vi "findCom.vi"(8 "error in (no error)":errorcluster, 11 "GiaoTiep in":refnum<class "GiaoTiepUART.lvclass">) -> (0 "error out":errorcluster, 3 "GiaoTiep out":refnum<class "GiaoTiepUART.lvclass">)   [LabVIEW 2014, in "LibraryGcode.lvlib" / "GiaoTiepUART.lvclass"]
uses:
  libraryGcode/ClassUART/GiaoTiepUART.lvclass
  <vilib>/Instr/_visa.llb/VISA Find Search Mode.ctl
  libraryGcode/ClassUART/GiaoTiepUART.lvclass/GiaoTiepUART.ctl
  <vilib>/Instr/_visa.llb/VISA Configure Serial Port (Instr).vi
panel:
  out "read buffer":string
  out "error out 2":errorcluster
  in  "termination char\n(0xA = '\\n' = LF)":u8=10 format="%.0x"
  out "StateError":bool
  out "OUT COM":refnum<visa-resource-name>
  out "CONNECT OK":bool
  out "find list":string[](array[string])
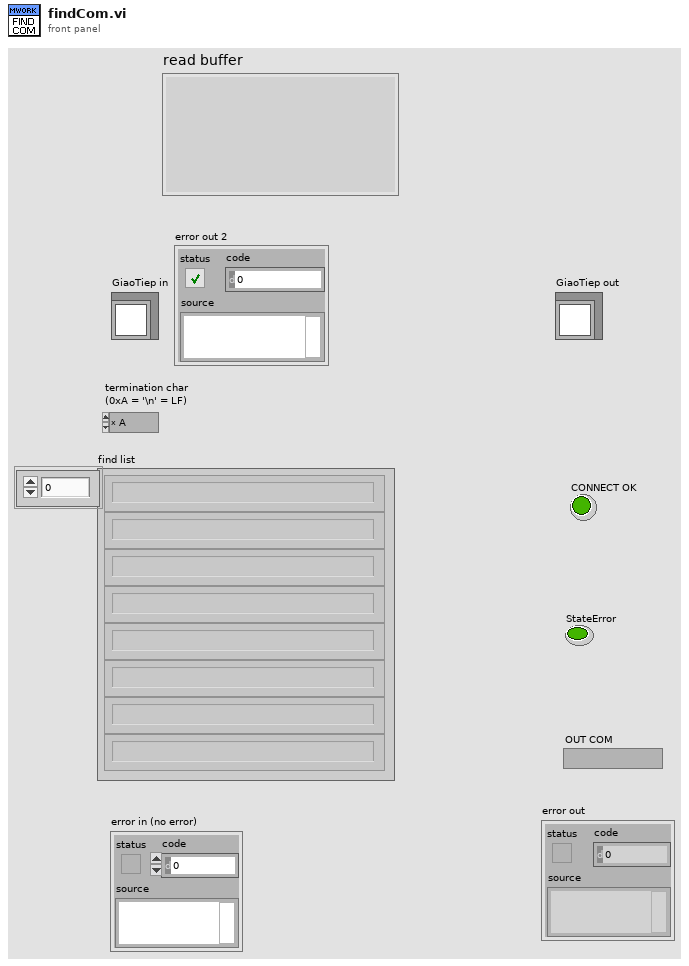
[diagram p1: front panel]
types:
  T1 = enum16{"InitCOM", "WriteCheck", "ReadCheck", "Comparedata", "End", "Stop"}
  T2 = typedef "VISA Find Search Mode.ctl" = u32
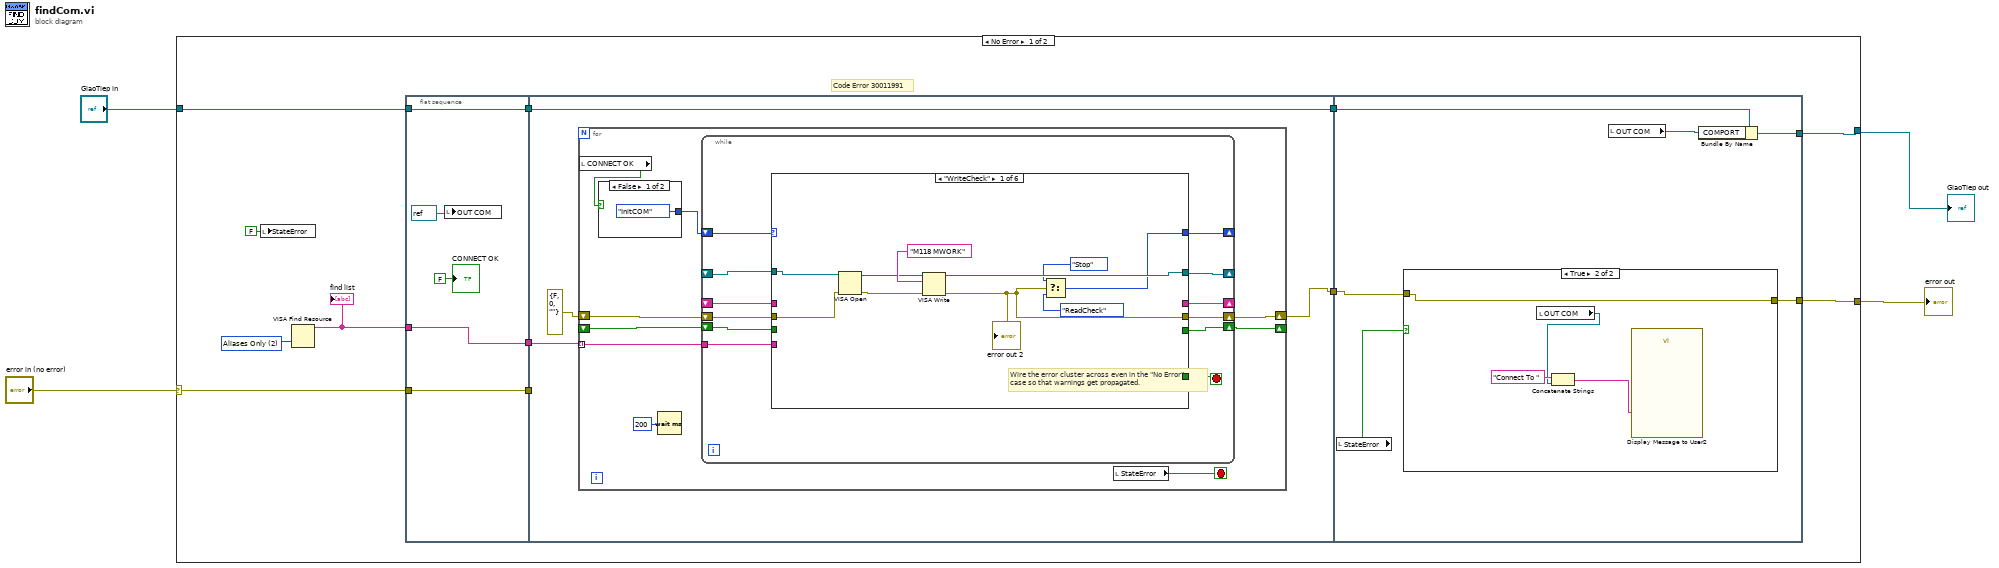
[diagram p0: block diagram]
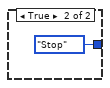
[diagram p2: hidden frame]
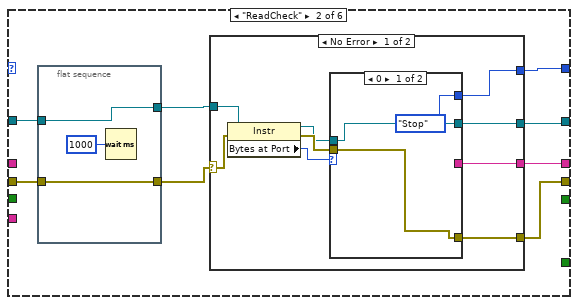
[diagram p3: hidden frame]
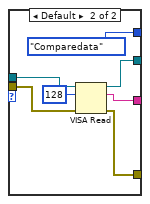
[diagram p4: hidden frame]
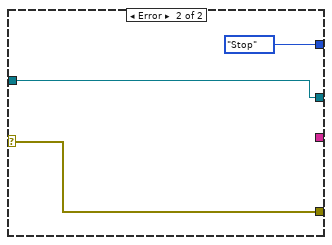
[diagram p5: hidden frame]
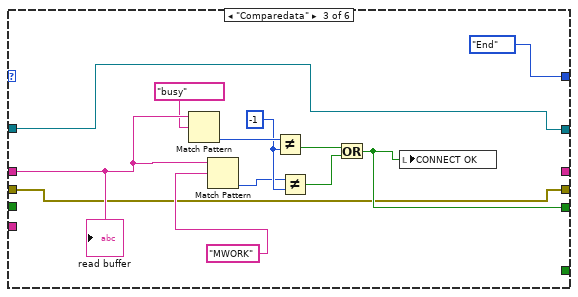
[diagram p6: hidden frame]
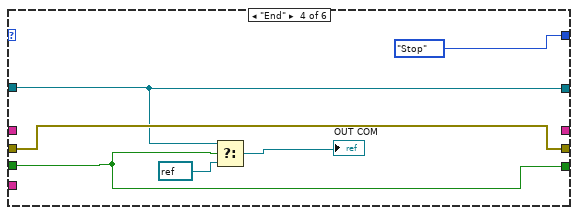
[diagram p7: hidden frame]
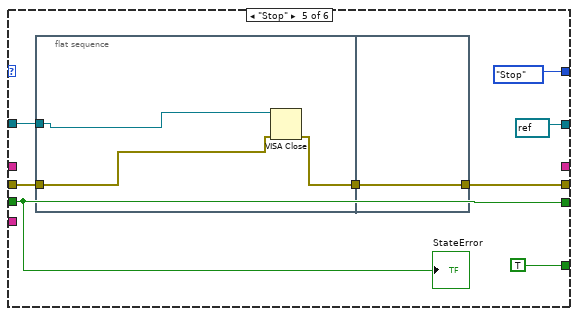
[diagram p8: hidden frame]
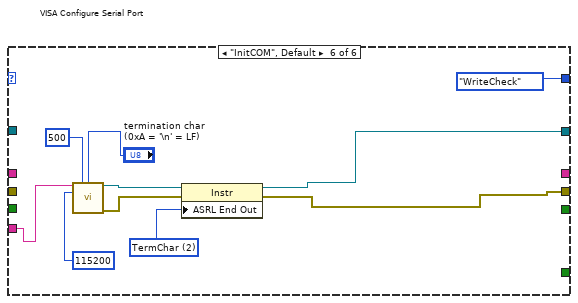
[diagram p9: hidden frame]
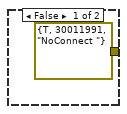
[diagram p10: hidden frame]
diagram:
  n1 = case shown="No Error" "error in (no error)" {
    selector: "error in (no error)" -> [w10 w144]
    tunnel: [w9 w144] -> w3
    tunnel: [w5 w143] -> w1
    tunnel: "GiaoTiep in" -> [w7 w143]
    frame No Error {
      w13 = T2 2 items=["Canonical Names Only"=0, "Aliases Only"=2, "Include Matching Aliases"=3, "Include All Aliases"=4] ("Search Mode")
      # "Code Error 30011991"
      # "Wire the error cluster across even in the \"No Error\"\ncase so that warnings get propagated."
      n2 = local write "StateError"(FALSE ("Boolean")) -> ()
      n3 = VISA Find Resource(10:w13) -> (3:w12:string[])  [unwired: 2 in, 2 out]
      "find list" <- w12
      n4 = flat-sequence {
        tunnel: w10 -> [w20]
        tunnel: w12 -> [w21]
        tunnel: [w21] -> w16
        tunnel: [w20] -> w15
        tunnel: [w17] -> w8
        tunnel: w7 -> [w17]
        tunnel: [w23] -> w14
        tunnel: w16 -> [w22]
        tunnel: w15 -> [_]
        tunnel: w8 -> [w24]
        tunnel: [w24] -> w6
        tunnel: w14 -> [w136]
        tunnel: [w135] -> w9
        tunnel: w6 -> [w134]
        tunnel: [w132] -> w5
        frame #0 {
          n5 = local write "OUT COM"(refnum<visa-resource-name> refnum ("f")) -> ()
          "CONNECT OK" <- FALSE ("CONNECT OK")
        }
        frame #1 {
          n6 = for {
            tunnel: w22 -> [w33] mode=indexing
            shift-right: [w28] -> _
            shift-left: _ -> [w29]
            shift-right: [w34] -> w23
            shift-left: errorcluster {"status"=FALSE, "code"=0, "source"=""} ("error out") -> [w32]
            stop <- w30 stop-if-true
            n7 = local read "CONNECT OK"() -> (w27:bool)
            n8 = case shown="False" w27 {
              tunnel: [T1."InitCOM" ("State") T1."Stop" ("State")] -> w26
              frame False {
              }
              frame True {
              }
            }
            n9 = Wait (ms)(milliseconds to wait=u32 200) -> ()  [unwired: 1 out]
            n10 = while {
              shift-right: [w38] -> _
              shift-left: w26 -> [w48]
              shift-right: [w40] -> _
              shift-left: _ -> [w47]
              shift-right: [w45] -> w34
              shift-left: w32 -> [w46]
              shift-right: [w44] -> _
              shift-left: _ -> [w43]
              shift-right: [w42] -> w28
              shift-left: w29 -> [w41]
              tunnel: w33 -> [w37]
              stop <- w39 stop-if-true
              n11 = case shown="\"WriteCheck\"" w48 {
                tunnel: w47 -> [w49 w61 w95 w104 w114 _]
                tunnel: [w58 w65 w95 w104 refnum<visa-resource-name> refnum ("VISA resource name out") w123] -> w40
                tunnel: w46 -> [w56 w60 w92 w108 w115 _]
                tunnel: [w50 w66 w92 w108 w116 w122] -> w45
                tunnel: [_ w64 _ _ _ _] -> w44
                tunnel: w43 -> [_ _ w101 _ _ _]
                tunnel: [_ _ w93 w107 w111 _] -> w42
                tunnel: w41 -> [_ _ _ w107 w111 _]
                tunnel: [_ _ _ _ TRUE _] -> w39
                tunnel: [w53 w63 T1."End" ("State") T1."Stop" ("State") T1."Stop" ("State") T1."WriteCheck" ("State")] -> w38
                tunnel: w37 -> [_ _ _ _ _ w124]
                frame "WriteCheck" {
                  n12 = VISA Open(error in (no error)=w56, VISA resource name=w49) -> (VISA resource name=w54:refnum<visa-resource-name>, error out=w55:errorcluster)  [unwired: 3 in]
                  n13 = VISA Write(VISA resource name=w54, write buffer="M118 MWORK" ("string"), error in (no error)=w55) -> (VISA resource name out=w58:refnum<visa-resource-name>, error out=w50:errorcluster)  [unwired: 1 out]
                  "error out 2" <- w50
                  n14 = Select(t=T1."Stop" ("f"), s=w50, f=T1."ReadCheck" ("State")) -> (s? t:f=w53:T1)
                }
                frame "ReadCheck" {
                  n15 = flat-sequence {
                    tunnel: [w69] -> w62
                    tunnel: w61 -> [w69]
                    tunnel: [w68] -> w59
                    tunnel: w60 -> [w68]
                    frame #0 {
                      n16 = Wait (ms)(milliseconds to wait=u32 1000) -> ()  [unwired: 1 out]
                    }
                  }
                  n17 = case shown="No Error" w59 {
                    selector: w59 -> [w70 w89]
                    tunnel: [w74 w89] -> w66
                    tunnel: w62 -> [w78 w90]
                    tunnel: [w75 w90] -> w65
                    tunnel: [w73 _] -> w64
                    tunnel: [w72 T1."Stop" ("State")] -> w63
                    frame No Error {
                      n18 = property class="Instr"(reference=w78, error in=w70) -> (reference out=w76:refnum<visa-resource-name>, error out=w77:errorcluster, "Bytes at Port"=w71:u32)
                      n19 = case shown="0" w71 {
                        tunnel: w77 -> [w79 w88]
                        tunnel: w76 -> [w80 w87]
                        tunnel: [w80 w86] -> w75
                        tunnel: [w79 w85] -> w74
                        tunnel: [_ w84] -> w73
                        tunnel: [T1."Stop" ("State") T1."Comparedata" ("State")] -> w72
                        frame 0 {
                        }
                        frame Default {
                          n20 = VISA Read(VISA resource name=w87, byte count=u32 128, error in (no error)=w88) -> (VISA resource name out=w86:refnum<visa-resource-name>, read buffer=w84:string, error out=w85:errorcluster)  [unwired: 1 out]
                        }
                      }
                    }
                    frame Error {
                    }
                  }
                }
                frame "Comparedata" {
                  w98 = -1 ("y")
                  n21 = Match Pattern(string=w101, regular expression="busy") -> (offset past match=w99:i32)  [unwired: 1 in, 3 out]
                  n22 = Match Pattern(string=w101, regular expression="MWORK" ("search string")) -> (offset past match=w94:i32)  [unwired: 1 in, 3 out]
                  n23 = Not Equal?(x=w99, y=w98) -> (x != y?=w97:bool)
                  n24 = Not Equal?(x=w94, y=w98) -> (x != y?=w96:bool)
                  n25 = Or(x=w97, y=w96) -> (x .or. y?=w93:bool)
                  n26 = local write "CONNECT OK"(w93) -> ()
                  "read buffer" <- w101
                }
                frame "End" {
                  n27 = Select(t=w104, s=w107, f=refnum<visa-resource-name> refnum) -> (s? t:f=→"OUT COM":refnum<visa-resource-name>)
                }
                frame "Stop" {
                  n28 = flat-sequence {
                    tunnel: w115 -> [w118]
                    tunnel: w114 -> [w119]
                    tunnel: [w120] -> w112
                    tunnel: [w121] -> w116
                    tunnel: w112 -> [w121]
                    frame #0 {
                      n29 = VISA Close(VISA resource name=w119, error in (no error)=w118) -> (error out=w120:errorcluster)
                    }
                    frame #1 {
                    }
                  }
                  "StateError" <- w111
                }
                frame "InitCOM", Default {
                  w130 = u16 2 items=["None", "Last Bit", "TermChar", "Break"] ("Serial Settings:End Mode for Writes")
                  n30 = call-poly "VISA Configure Serial Port"("VISA resource name"=w124, "timeout (10sec)"=u32 500, "termination char\n(0xA = '\\n' = LF)"="termination char\n(0xA = '\\n' = LF)", "baud rate (9600)"=u32 115200) -> ("VISA resource name out"=w128:refnum<visa-resource-name>, "error out"=w129:errorcluster)  [unwired: 10 in]
                  n31 = property class="Instr"(reference=w128, error in=w129, "ASRL End Out"=w130) -> (reference out=w123:refnum<visa-resource-name>, error out=w122:errorcluster)
                }
              }
            }
            n32 = local read "StateError"() -> (w30:bool)
          }
        }
        frame #2 {
          n33 = local read "StateError"() -> (w137:bool)
          n34 = case shown="True" w137 {
            tunnel: w136 -> [_ w139]
            tunnel: [errorcluster {"status"=TRUE, "code"=30011991, "source"="NoConnect "} ("error out") w139] -> w135
            frame False {
            }
            frame True {
              n35 = local read "OUT COM"() -> (w140:refnum<visa-resource-name>)
              n36 = Concatenate Strings("Connect To " ("string"), w140) -> (w142:string)
              n37 = call "Display Message to User2"("Message"=w142) -> ()  [unwired: 9 in, 2 out]
            }
          }
          n38 = local read "OUT COM"() -> (w133:refnum<visa-resource-name>)
          n39 = Bundle By Name(cluster=w134, "COMPORT"=w133) -> (w132:refnum<class "GiaoTiepUART.lvclass">)
        }
      }
    }
    frame Error {
    }
  }
  "error out" <- w3
  "GiaoTiep out" <- w1
